vi "saveSignalToCSV(SubVI).vi"(1 "název souboru":string, 2 "Graf pro porovnání signálu":waveform(dbl)[](array[waveform])) -> ()   [LabVIEW 2025]
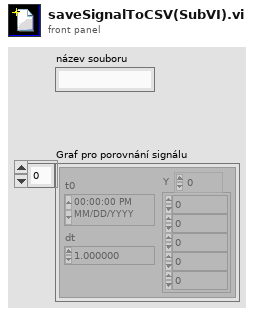
[diagram p1: front panel]
types:
  T1 = enum16{"open", "replace", "create", "open or create", "replace or create", "replace or create with confirmation"}
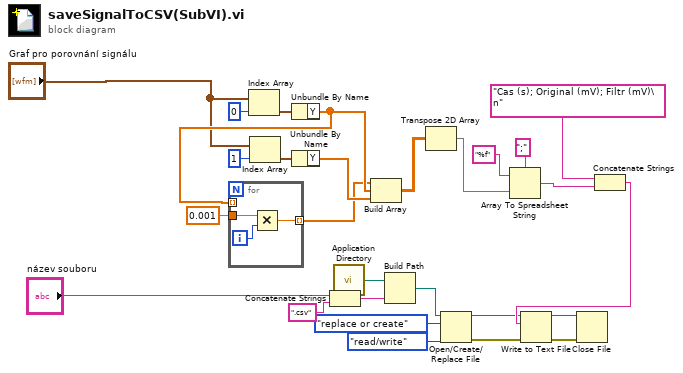
[diagram p0: block diagram]
diagram:
  n1 = Index Array(array="Graf pro porovnání signálu", index=0) -> (element=w18:waveform(dbl))
  n2 = Index Array(array="Graf pro porovnání signálu", index=1) -> (element=w21:waveform(dbl))
  n3 = Unbundle By Name(w18) -> ("Y"=w27:dbl[])
  n4 = for {
    tunnel: 0.001 -> [w30]
    tunnel: [w28] -> w25 mode=indexing
    tunnel: w27 -> [_] mode=indexing
    i -> [w29]
    n5 = Multiply(x=w30, y=w29) -> (x*y=w28:dbl)
  }
  n6 = Unbundle By Name(w21) -> ("Y"=w26:dbl[])
  n7 = Concatenate Strings("název souboru", ".csv") -> (w13:string)
  n8 = call <vilib>:"Application Directory.vi"() -> ("Application Directory"=w11:path)
  n9 = Build Array(w25, w27, w26) -> (w23:dbl[][])
  n10 = Build Path(base path=w11, name or relative path=w13) -> (appended path=w14:path)
  n11 = Transpose 2D Array(2D array=w23) -> (transposed array=w24:dbl[][])
  n12 = Open/Create/Replace File(file path (use dialog)=w14, operation (0:open)=T1."replace or create", access (0:read/write)=enum16{"read/write", "read-only", "write-only"}."read/write") -> (refnum out=w7:refnum<file>, error out=w5:errorcluster)  [unwired: 3 in, 1 out]
  n13 = Array To Spreadsheet String(delimiter (Tab)=";", array=w24, 3:"%f" ("format string")) -> (spreadsheet string=w3:string)
  n14 = Concatenate Strings("Cas (s); Original (mV); Filtr (mV)\n" ("string"), w3) -> (w15:string)
  n15 = Write to Text File(file (use dialog)=w7, text=w15, error in=w5) -> (refnum out=w8:refnum<file>, error out=w6:errorcluster)  [unwired: 1 in, 1 out]
  n16 = Close File(refnum=w8, error in=w6) -> ()  [unwired: 2 out]
